vi "Thermocouple(MCP9600).vi"() -> ()   [LabVIEW 2024]
uses:
  ThermocoupleType.ctl
  Driver/Public/Digital Pull Direction.ctl
  4d20a38f-85d9-49a3-8b57-4ea18b2081fb.vi
  e936b299-2736-4eae-a5ba-62d121779c0d.vi
  Driver/CTIPicoVISA.lvlib
panel:
  in  "Stop":bool
  out "Thermometer":dbl(slide) scale=0.0..1000.0
  out "Array":string[](array[string])
  out "DeviceID":string
  in  "Thermocouple Type":T1
  out "Temperature":dbl(graph)
  in  "Grove Connector":enum16{"I2C0", "I2C1"}(ring)
  in  "VISA resource name in":refnum<visa-resource-name>="COM10"
  out "LoopIndex":i32
  out "Identity":T2
  # "https://wiki.seeedstudio.com/Grove-I2C_Thermocouple_Amplifier-MCP9600/"
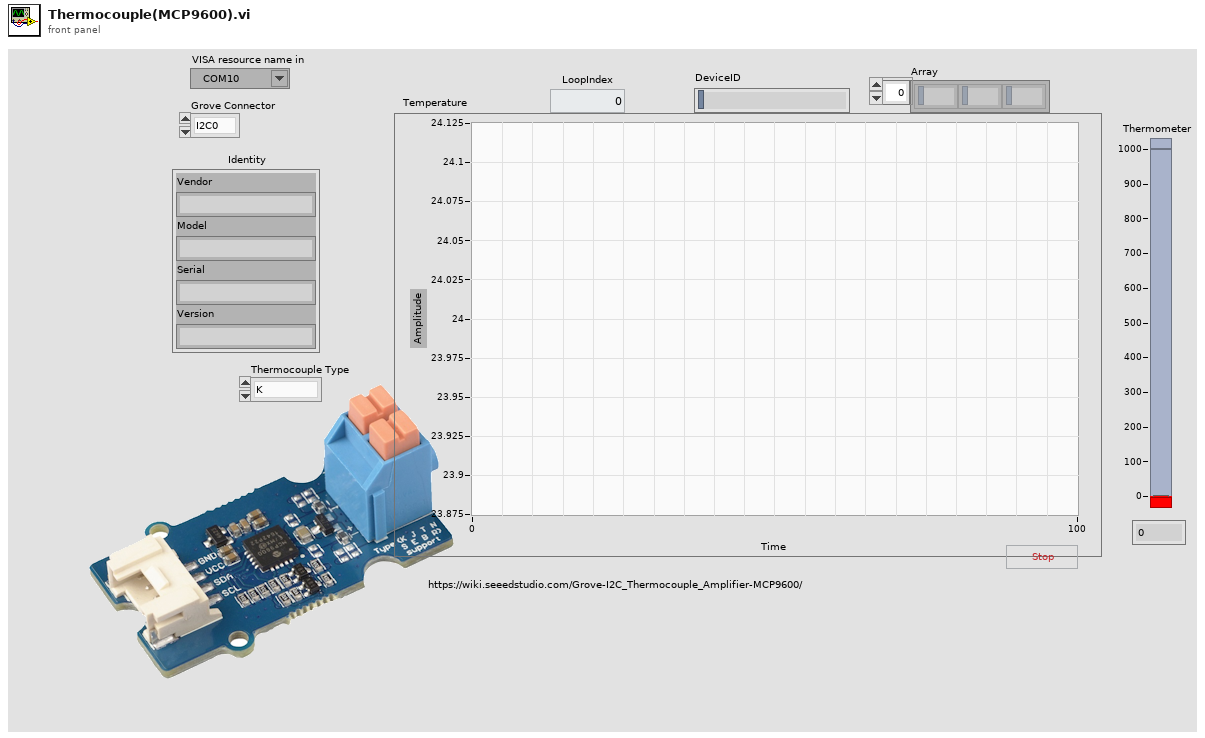
[diagram p1: front panel]
types:
  T1 = typedef "ThermocoupleType.ctl" = enum16{"K", "J", "T", "N", "S", "E", "B", "R"}
  T2 = cluster{"Vendor":string, "Model":string, "Serial":string, "Version":string}
  T3 = typedef "CTIPicoVISA.lvlib/Digital Pull Direction.ctl" = enum16{"None", "Up", "Down", "Both"}
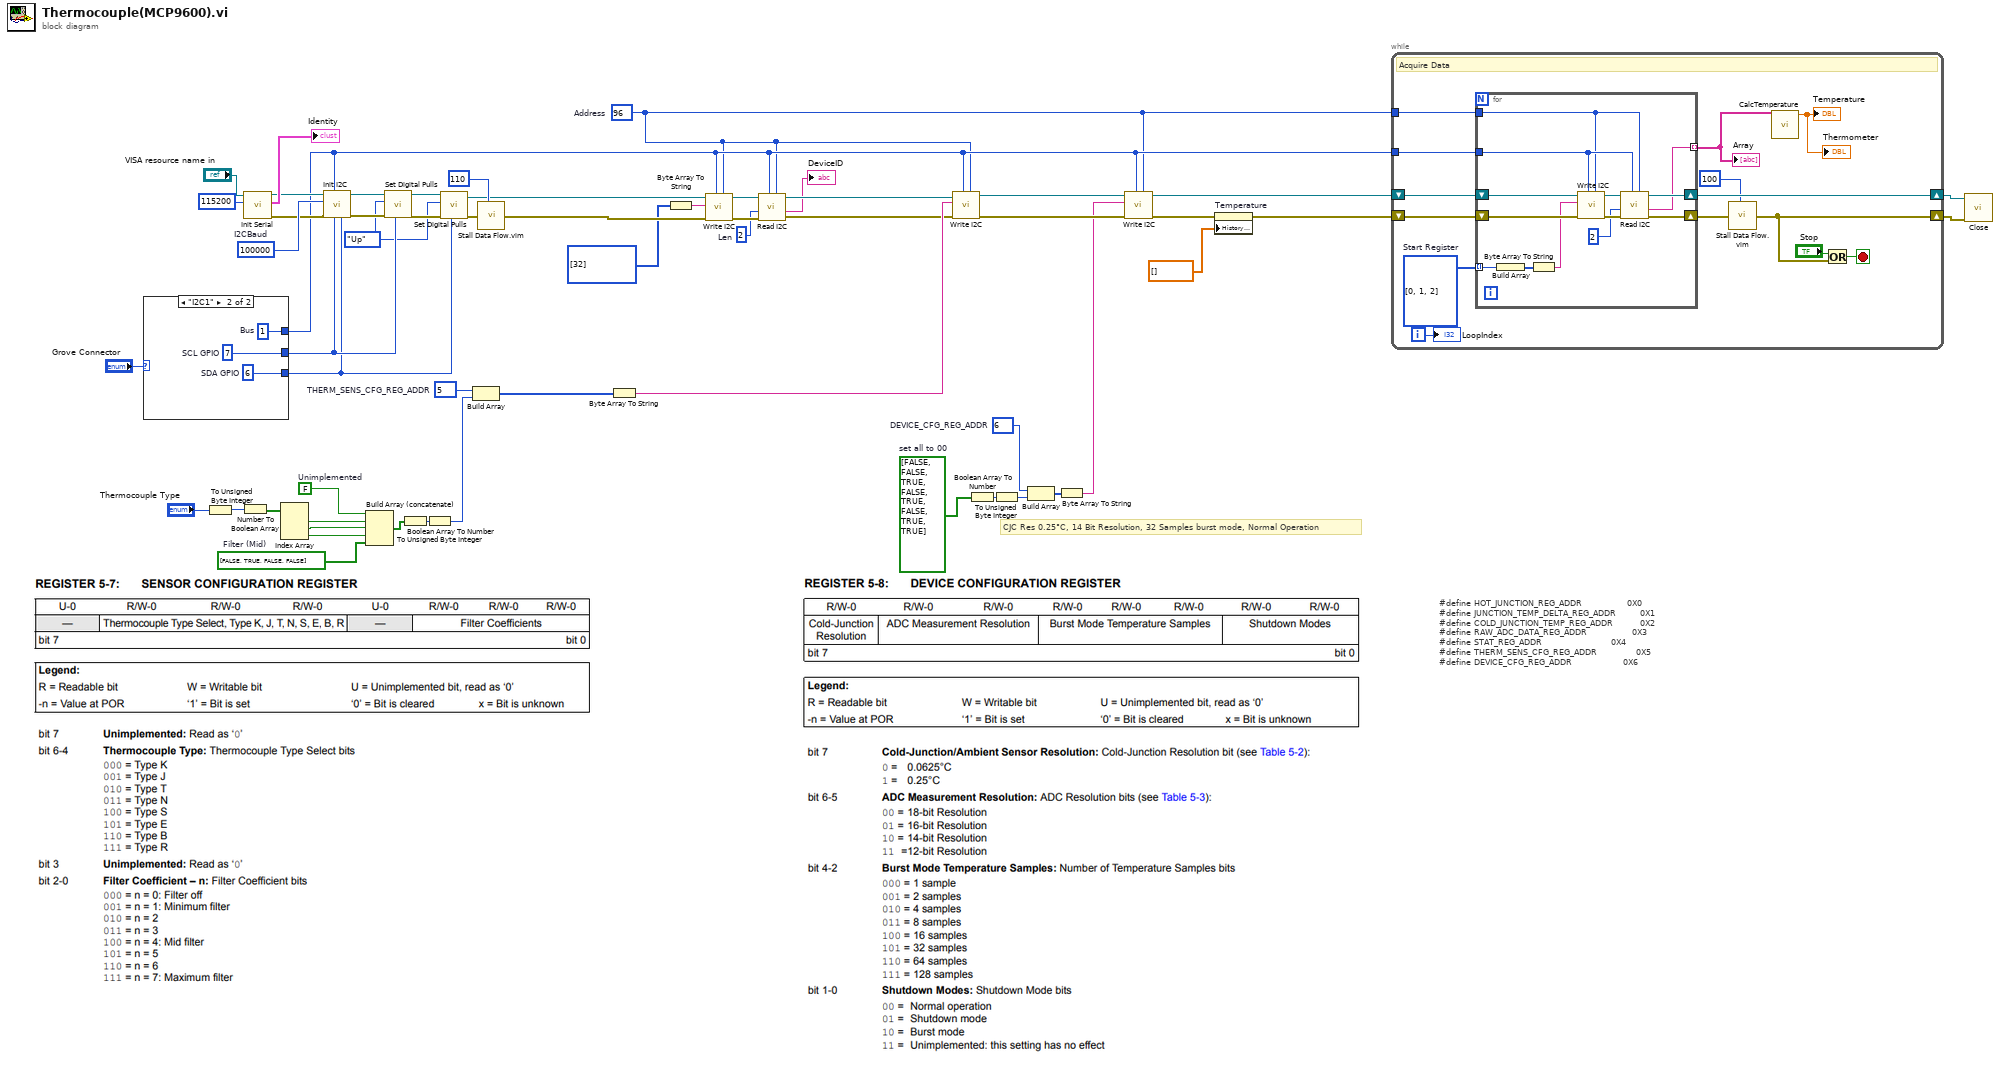
[diagram p0: block diagram]
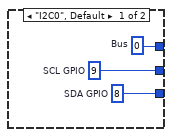
[diagram p2: hidden frame]
diagram:
  w3 = u8 2  # Len
  w1 = u8 96  # Address
  w18 = u8 6  # DEVICE_CFG_REG_ADDR
  w20 = bool[] [FALSE, FALSE, TRUE, FALSE, TRUE, FALSE, TRUE, TRUE]  # set all to 00
  w13 = bool[] [FALSE, TRUE, FALSE, FALSE]  # Filter (Mid)
  w27 = FALSE  # Unimplemented
  w45 = Digital_Pull_Direction."Up" ("Pull")
  w52 = u32 100000  # I2CBaud
  w56 = u8 5  # THERM_SENS_CFG_REG_ADDR
  # "CJC Res 0.25°C, 14 Bit Resolution, 32 Samples burst mode, Normal Operation"
  # "#define HOT_JUNCTION_REG_ADDR               0X0\n#define JUNCTION_TEMP_DELTA_REG_ADDR        0X1\n#define COLD_JUNCTION_TEMP_REG_ADDR         0X2\n#define RAW_ADC_DATA_REG_ADDR               0X3\n#define STAT_REG_ADDR                       0X4\n#define THERM_SENS_CFG_REG_ADDR             0X5\n#define DEVICE_CFG_REG_ADDR                 0X6"
  n1 = case shown="\"I2C1\"" "Grove Connector" {
    tunnel: [w59 w62] -> w46
    tunnel: [w58 w61] -> w44
    tunnel: [w57 w60] -> w10
    frame "I2C0", Default {
      w57 = u8 0  # Bus
      w58 = 8  # SDA GPIO
      w59 = 9  # SCL GPIO
    }
    frame "I2C1" {
      w60 = u8 1  # Bus
      w61 = 6  # SDA GPIO
      w62 = 7  # SCL GPIO
    }
  }
  n2 = To Unsigned Byte Integer(number="Thermocouple Type") -> (unsigned 8bit integer=w33:u8)
  n3 = Number To Boolean Array(number=w33) -> (Boolean array=w31:bool[])
  n4 = call "Init Serial.vi"("Baud (115200)"=u32 115200, "VISA resource name in"="VISA resource name in") -> ("error out"=w40:errorcluster, "Identity"=→"Identity":T2, "VISA resource name Out"=w41:refnum<visa-resource-name>)  [unwired: 7 in]
  n5 = Index Array(array=w31) -> (element #1=w30:bool, element #2=w29:bool, element #3=w28:bool)  [unwired: 3 in]
  n6 = call "Init I2C.vi"("SDA GPIO"=w44, "SCL GPIO"=w46, "Bus"=w10, "error in (no error)"=w40, "Baud"=w52, "VISA resource name in"=w41) -> ("error out"=w49:errorcluster, "VISA resource name"=w50:refnum<visa-resource-name>)  [unwired: 4 in]
  n7 = Build Array (concatenate)(w27, w30, w29, w28, w13) -> (w26:bool[])
  n8 = call "Set Digital Pulls.vi"("GPIO"=w46, "error in (no error)"=w49, "Pull"=w45, "VISA resource name in"=w50) -> ("error out"=w47:errorcluster, "VISA resource name"=w48:refnum<visa-resource-name>)  [unwired: 6 in]
  n9 = Boolean Array To Number(Boolean array=w26) -> (number=w25:u32)
  n10 = To Unsigned Byte Integer(number=w25) -> (unsigned 8bit integer=w24:u8)
  n11 = call "Set Digital Pulls.vi"("GPIO"=w44, "error in (no error)"=w47, "Pull"=w45, "VISA resource name in"=w48) -> ("error out"=w42:errorcluster, "VISA resource name"=w11:refnum<visa-resource-name>)  [unwired: 6 in]
  n12 = Build Array(w56, w24) -> (w55:u8[])
  n13 = call "Stall Data Flow.vim"("value in"=w42, "milliseconds to wait"=u32 110) -> ("value out"=w12:errorcluster)  [unwired: 1 out]
  n14 = Byte Array To String(unsigned byte array=w55) -> (string=w35:string)
  n15 = Byte Array To String(unsigned byte array=u8[] [32] ("Start Register")) -> (string=w6:string)
  n16 = call "Write I2C.vi"("Address"=w1, "Bus"=w10, "error in (no error)"=w12, "Data"=w6, "VISA resource name in"=w11) -> ("error out"=w5:errorcluster, "VISA resource name"=w4:refnum<visa-resource-name>)  [unwired: 5 in]
  n17 = call "Read I2C.vi"("Address"=w1, "Bus"=w10, "error in (no error)"=w5, "Len"=w3, "VISA resource name in"=w4) -> ("error out"=w8:errorcluster, "Data"=→"DeviceID":string, "VISA resource name"=w9:refnum<visa-resource-name>)  [unwired: 4 in]
  n18 = call "Write I2C.vi"("Address"=w1, "Bus"=w10, "error in (no error)"=w8, "Data"=w35, "VISA resource name in"=w9) -> ("error out"=w22:errorcluster, "VISA resource name"=w23:refnum<visa-resource-name>)  [unwired: 5 in]
  n19 = Boolean Array To Number(Boolean array=w20) -> (number=w21:u32)
  n20 = To Unsigned Byte Integer(number=w21) -> (unsigned 8bit integer=w19:u8)
  n21 = Build Array(w18, w19) -> (w17:u8[])
  n22 = Byte Array To String(unsigned byte array=w17) -> (string=w16:string)
  n23 = call "Write I2C.vi"("Address"=w1, "Bus"=w10, "error in (no error)"=w22, "Data"=w16, "VISA resource name in"=w23) -> ("error out"=w15:errorcluster, "VISA resource name"=w14:refnum<visa-resource-name>)  [unwired: 5 in]
  n24 = property on="Temperature" class="WFChart (strict)"(error in=w15, "History Data"=dbl[] []) -> (error out=w34:errorcluster)  [unwired: 1 in, 1 out]
  n25 = while {
    tunnel: w10 -> [w70]
    tunnel: w1 -> [w69]
    shift-right: [w65] -> w38
    shift-left: w34 -> [w76]
    shift-right: [w68] -> w39
    shift-left: w14 -> [w75]
    i -> [w73]
    stop <- w72 stop-if-true
    w71 = u8[] [0, 1, 2]  # Start Register
    # "Acquire Data"
    n26 = for {
      tunnel: w71 -> [w83] mode=indexing
      tunnel: w70 -> [w82]
      tunnel: w69 -> [w81]
      shift-right: [w79] -> w67
      shift-left: w76 -> [w89]
      shift-right: [w80] -> w68
      shift-left: w75 -> [w88]
      tunnel: [w78] -> w66 mode=indexing
      n27 = Build Array(w83) -> (w77:u8[])
      n28 = Byte Array To String(unsigned byte array=w77) -> (string=w87:string)
      n29 = call "Write I2C.vi"("Address"=w81, "Bus"=w82, "error in (no error)"=w89, "Data"=w87, "VISA resource name in"=w88) -> ("error out"=w86:errorcluster, "VISA resource name"=w85:refnum<visa-resource-name>)  [unwired: 5 in]
      n30 = call "Read I2C.vi"("Address"=w81, "Bus"=w82, "error in (no error)"=w86, "Len"=u8 2 ("Read Len"), "VISA resource name in"=w85) -> ("error out"=w79:errorcluster, "Data"=w78:string, "VISA resource name"=w80:refnum<visa-resource-name>)  [unwired: 4 in]
    }
    "Array" <- w66
    n31 = call "Stall Data Flow.vim"("value in"=w67, "milliseconds to wait"=u32 100) -> ("value out"=w65:errorcluster)  [unwired: 1 out]
    n32 = call "CalcTemperature.vi"("Array"=w66) -> ("HJ Temperature (°C)"=→"Temperature" →"Thermometer":dbl)  [unwired: 10 in]
    n33 = Or(x="Stop", y=w65) -> (x .or. y?=w72:bool)
    "LoopIndex" <- w73
  }
  n34 = call "Close.vi"("error in (no error)"=w38, "VISA resource name in"=w39) -> ()  [unwired: 9 in, 1 out]
